vi "New Verify as JSON.vi"(8 "error in":errorcluster, 11 "TestCase in":refnum<class "TestCase.lvclass">) -> (0 "error out":errorcluster, 3 "TestCase out":refnum<class "TestCase.lvclass">)   [LabVIEW 2025, in "VITester.Extension.lvlib"]
uses:
  VITester.Extension.lvlib
  <vilib>/Addons/_JKI Toolkits/VI Tester/TestCase.llb/TestCase.lvclass
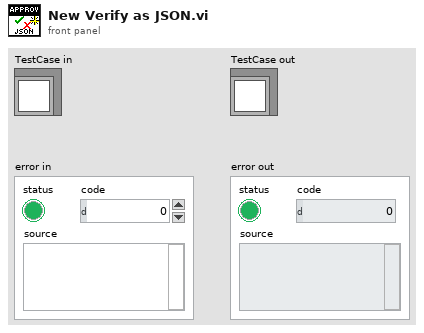
[diagram p1: front panel]
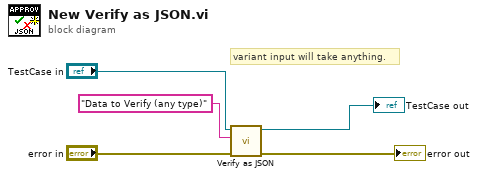
[diagram p0: block diagram]
diagram:
  # "variant input will take anything."
  n1 = call "Verify as JSON.vi"("error in"="error in", "Anything"="Data to Verify (any type)", "TestCase in"="TestCase in") -> ("error out"=→"error out":errorcluster, "TestCase out"=→"TestCase out":refnum<class "TestCase.lvclass">)  [unwired: 7 in]
